vi "恒流源控制.vi"   [LabVIEW 2012]
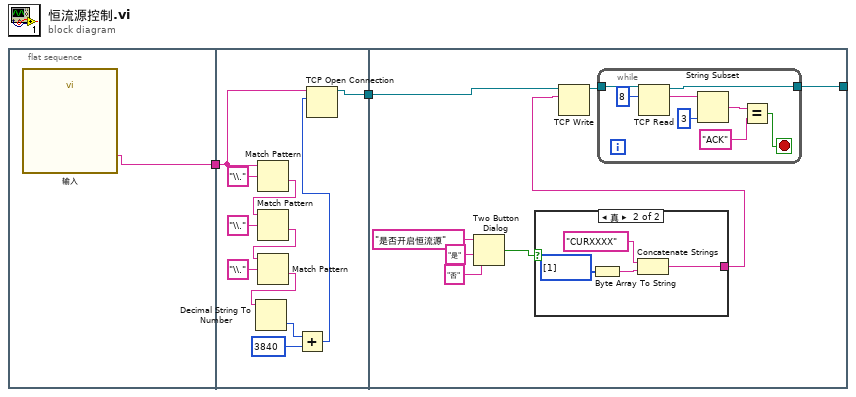
[diagram p0: block diagram]
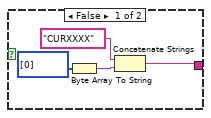
[diagram p2: hidden frame]
diagram:
  n1 = flat-sequence {
    tunnel: [w3] -> w2
    tunnel: [w14] -> w1
    tunnel: w2 -> [w8]
    tunnel: w1 -> [w22]
    tunnel: [w20] -> _
    frame #0 {
      n2 = call "输入"() -> ("IP地址"=w3:string)  [unwired: 17 in, 2 out]
    }
    frame #1 {
      n3 = Match Pattern(string=w8, regular expression="\\." ("正则表达式")) -> (after substring=w10:string)  [unwired: 1 in, 3 out]
      n4 = Match Pattern(string=w10, regular expression="\\." ("正则表达式")) -> (after substring=w9:string)  [unwired: 1 in, 3 out]
      n5 = Match Pattern(string=w9, regular expression="\\." ("正则表达式")) -> (after substring=w7:string)  [unwired: 1 in, 3 out]
      n6 = Decimal String To Number(string=w7) -> (number=w6:i32)  [unwired: 2 in, 1 out]
      n7 = Add(x=w6, y=3840) -> (x+y=w4:i32)
      n8 = TCP Open Connection(address=w8, remote port or service name=w4) -> (connection ID=w14:refnum<k5>)  [unwired: 3 in, 1 out]
    }
    frame #2 {
      n9 = Two Button Dialog(message="是否开启恒流源" ("消息"), 1:"否" ("F按钮名称（“取消”）"), 2:"是" ("T按钮名称（“确定”）")) -> (T button?=w19:bool)
      n10 = case shown="真" w19 {
        tunnel: [w23 w27] -> w15
        frame False {
          n11 = Byte Array To String(unsigned byte array=u8[] [0] ("无符号字节数组")) -> (string=w25:string)
          n12 = Concatenate Strings("CURXXXX" ("数据输入"), w25) -> (w23:string)
        }
        frame True {
          n13 = Byte Array To String(unsigned byte array=u8[] [1] ("无符号字节数组")) -> (string=w29:string)
          n14 = Concatenate Strings("CURXXXX" ("数据输入"), w29) -> (w27:string)
        }
      }
      n15 = TCP Write(connection ID=w22, data in=w15) -> (connection ID out=w21:refnum<k5>)  [unwired: 2 in, 2 out]
      n16 = while {
        tunnel: w21 -> [w38]
        tunnel: [w32] -> w20
        stop <- w33 stop-if-true
        n17 = TCP Read(connection ID=w38, bytes to read=8 ("读取的字节")) -> (connection ID out=w32:refnum<k5>, data out=w36:string)  [unwired: 3 in, 1 out]
        n18 = String Subset(string=w36, length (rest)=3 ("偏移量(0)")) -> (substring=w35:string)  [unwired: 1 in]
        n19 = Equal?(x=w35, y="ACK") -> (x = y?=w33:bool)
      }
    }
  }
